vi "ESP32_initialize_2.vi"(0 "ESP32 IN":refnum<visa-resource-name>, 1 "Switch On Time":u8 caption="Switch On Time(uS)", 2 "Switch Off Time":u8=100 caption="Switch Off Time(uS)", 3 "Enable Accurate \nMeasure":bool=TRUE, 5 "Sample Mode":u16(ring) items=["Normal", "Interlanced", "Serial", "Seperated Serial"], 11 "error in (no error)":errorcluster, 12 "Measure Current \nOnly":bool=TRUE, 13 "Sample Measure\nTime(uS)":i32=100, 14 "Sample number":i32=1) -> (4 "ESP32 out":refnum<visa-resource-name>, 15 "error out":errorcluster)   [LabVIEW 2023]
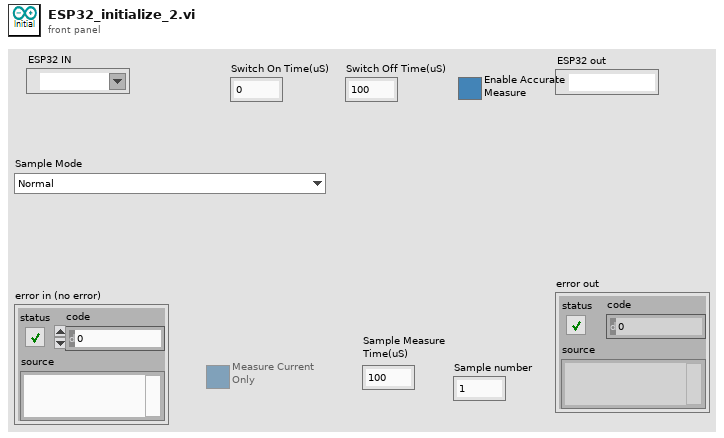
[diagram p1: front panel]
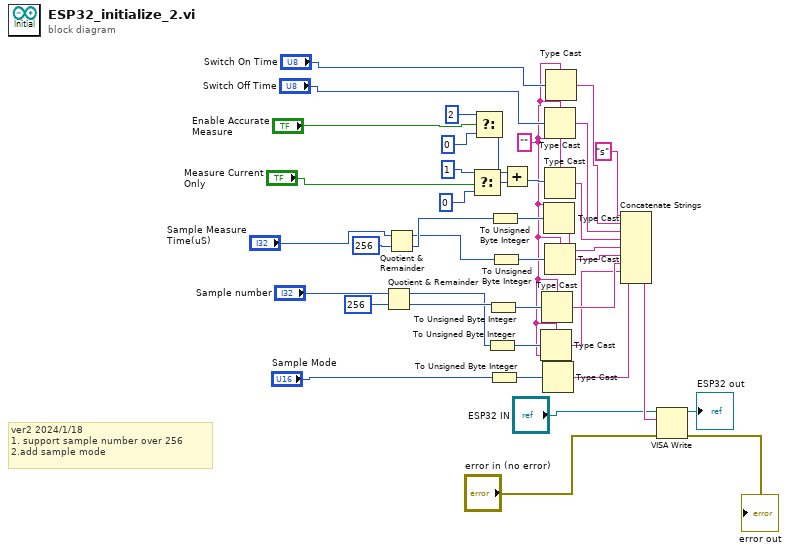
[diagram p0: block diagram]
diagram:
  w3 = "" ("string")
  # "ver2 2024/1/18\n1. support sample number over 256\n2.add sample mode"
  n1 = Quotient & Remainder(x="Sample number", y=256) -> (x-y*floor(x/y)=w6:i32, floor(x/y)=w10:i32)
  n2 = Quotient & Remainder(x="Sample Measure\nTime(uS)", y=u32 256) -> (x-y*floor(x/y)=w17:u32, floor(x/y)=w31:u32)
  n3 = Select(t=u8 1, s="Measure Current \nOnly", f=u8 0) -> (s? t:f=w28:u8)
  n4 = Select(t=u8 2, s="Enable Accurate \nMeasure", f=u8 0) -> (s? t:f=w29:u8)
  n5 = To Unsigned Byte Integer(number=w6) -> (unsigned 8bit integer=w7:u8)
  n6 = To Unsigned Byte Integer(number=w10) -> (unsigned 8bit integer=w12:u8)
  n7 = To Unsigned Byte Integer(number="Sample Mode") -> (unsigned 8bit integer=w4:u8)
  n8 = To Unsigned Byte Integer(number=w31) -> (unsigned 8bit integer=w35:u8)
  n9 = To Unsigned Byte Integer(number=w17) -> (unsigned 8bit integer=w39:u8)
  n10 = Add(x=w29, y=w28) -> (x+y=w27:u8)
  n11 = Type Cast(type=w3, x=w7) -> (*(type *) &x=w5:string)
  n12 = Type Cast(type=w3, x=w12) -> (*(type *) &x=w11:string)
  n13 = Type Cast(type=w3, x=w4) -> (*(type *) &x=w1:string)
  n14 = Type Cast(type=w3, x=w35) -> (*(type *) &x=w36:string)
  n15 = Type Cast(type=w3, x="Switch Off Time") -> (*(type *) &x=w23:string)
  n16 = Type Cast(type=w3, x=w27) -> (*(type *) &x=w37:string)
  n17 = Type Cast(type=w3, x=w39) -> (*(type *) &x=w40:string)
  n18 = Type Cast(type=w3, x="Switch On Time") -> (*(type *) &x=w24:string)
  n19 = Concatenate Strings("s" ("data in"), w24, w23, w37, w36, w40, w11, w5, w1) -> (w38:string)
  n20 = VISA Write(VISA resource name="ESP32 IN", write buffer=w38, error in (no error)="error in (no error)") -> (VISA resource name out=→"ESP32 out":refnum<visa-resource-name>, error out=→"error out":errorcluster)  [unwired: 1 out]
